vi "Instantiate Function [On Syntax].vi"(0 "function manager in":refnum<class "function manager.lvclass">, 5 "Function String":string, 11 "error in (no error)":errorcluster) -> (4 "function manager out":refnum<class "function manager.lvclass">, 6 "function obj":refnum<class "functionbase.lvclass">, 8 "Valid Syntax?":bool, 15 "error out":errorcluster)   [LabVIEW 2016, in "function manager.lvclass"]
uses:
  function manager.lvclass
  functionsbase/functionbase.lvclass
  function manager.lvclass/function manager.ctl
  functionsbase/functionbase.lvclass/functionbase.ctl
  functionsbase/properties/Write Func Syntax.vi
  functionsbase/properties/Write Func Full String.vi
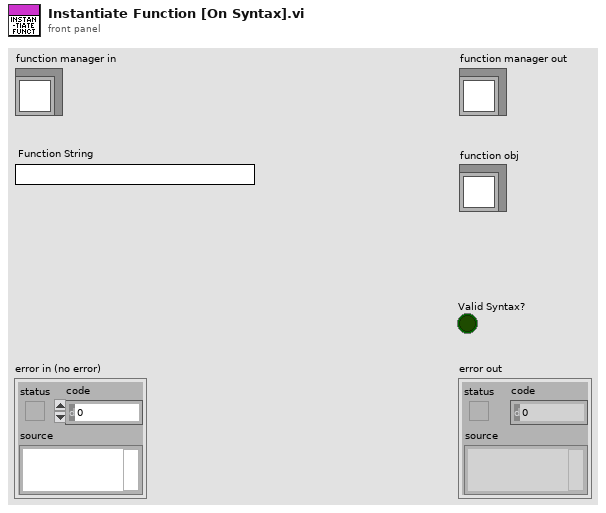
[diagram p1: front panel]
types:
  T1 = typedef "Scan Syntax Format.ctl" = cluster{"Syntax":string, "Variable#":i32, "Variables Name":string[]}
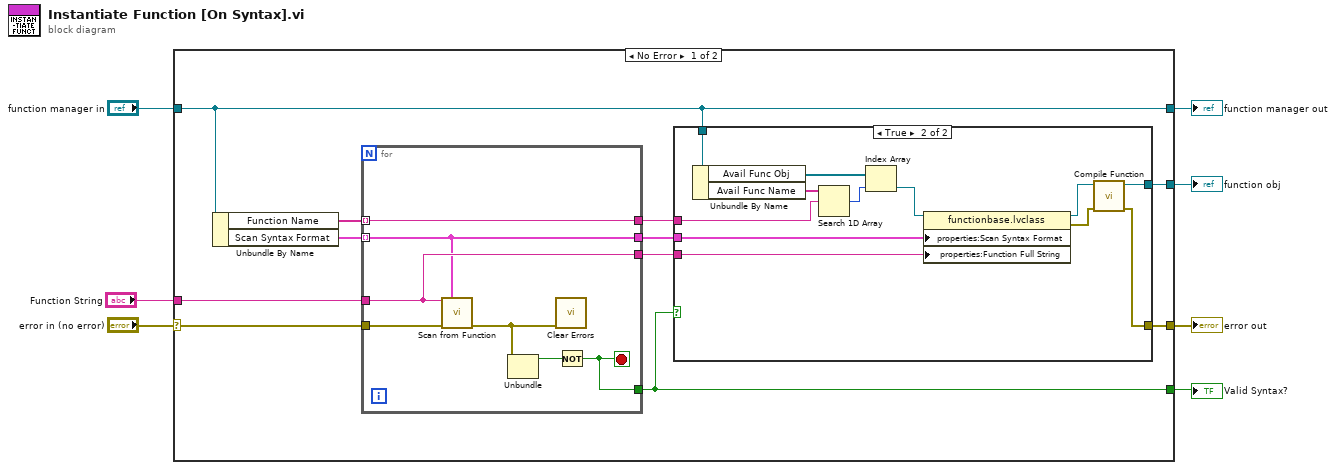
[diagram p0: block diagram]
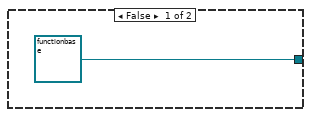
[diagram p2: hidden frame]
diagram:
  n1 = case shown="No Error" "error in (no error)" {
    selector: "error in (no error)" -> [w15 w40]
    tunnel: [w10 w40] -> w6
    tunnel: [w14 w39] -> w4
    tunnel: "function manager in" -> [w14 w39]
    tunnel: "Function String" -> [w18 _]
    tunnel: [w8 _] -> w2
    tunnel: [w9 _] -> w1
    frame No Error {
      n2 = Unbundle By Name(w14) -> ("Function Name"=w16:string[], "Scan Syntax Format"=w17:T1[])
      n3 = for {
        tunnel: w18 -> [w33]
        tunnel: w17 -> [w32] mode=indexing
        tunnel: w16 -> [w36] mode=indexing
        tunnel: w15 -> [w35]
        tunnel: [w37] -> w8
        tunnel: [w36] -> w13
        tunnel: [w32] -> w12
        tunnel: [w33] -> w11
        stop <- w37 stop-if-true
        n4 = call "Scan from Function.vi"("initial string"=w33, "Syntax Format"=w32, "error in"=w35) -> ("error out"=w34:errorcluster)  [unwired: 9 in, 3 out]
        n5 = Unbundle(w34) -> ("status"=w38:bool)  [unwired: 2 out]
        n6 = call <vilib>:"Clear Errors.vi"("error in (no error)"=w34) -> ()  [unwired: 5 in, 2 out]
        n7 = Not(x=w38) -> (.not. x?=w37:bool)
      }
      n8 = case shown="True" w8 {
        tunnel: w14 -> [_ w31]
        tunnel: w13 -> [_ w29]
        tunnel: w12 -> [_ w24]
        tunnel: w11 -> [_ w25]
        tunnel: [_ w20] -> w10
        tunnel: [refnum<class "functionbase.lvclass"> refnum ("functionbase.lvclass") w22] -> w9
        frame False {
        }
        frame True {
          n9 = Unbundle By Name(w31) -> ("Avail Func Obj"=w28:refnum<class "functionbase.lvclass">[], "Avail Func Name"=w30:string[])
          n10 = Search 1D Array(1D array=w30, element=w29) -> (index of element=w27:i32)  [unwired: 1 in]
          n11 = Index Array(array=w28, index=w27) -> (element=w26:refnum<class "functionbase.lvclass">)
          n12 = property class="functionbase.lvclass"(reference=w26, "properties:Scan Syntax Format"=w24, "properties:Function Full String"=w25) -> (reference out=w23:refnum<class "functionbase.lvclass">, error out=w21:errorcluster)  [unwired: 1 in]
          n13 = call-dynamic "Compile Function.vi"("error in (no error)"=w21, "functionbase in"=w23) -> ("error out"=w20:errorcluster, "functionbase out"=w22:refnum<class "functionbase.lvclass">)  [unwired: 8 in]
        }
      }
    }
    frame Error {
    }
  }
  "error out" <- w6
  "function manager out" <- w4
  "Valid Syntax?" <- w2
  "function obj" <- w1
